vi "文本文件（将100个正弦数据以3位小数的形式写入文本文件）.vi"() -> ()   [LabVIEW 2017]
panel:
  out "写入数据":dbl[](array[numeric])
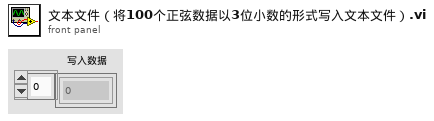
[diagram p1: front panel]
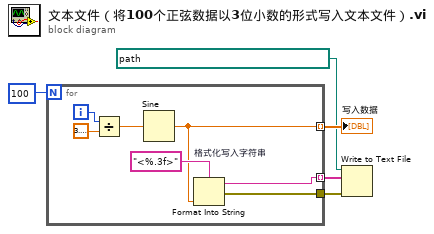
[diagram p0: block diagram]
diagram:
  n1 = for {
    N: 100 -> [_]
    tunnel: [w8] -> w4 mode=indexing
    tunnel: [w7] -> w3
    tunnel: [w6] -> w2 mode=indexing
    i -> [w12]
    n2 = Divide(x=w12, y=3.141592653589793) -> (x/y=w10:dbl)
    n3 = Sine(x=w10) -> (sin(x)=w6:dbl)
    n4 = Format Into String "格式化写入字符串"(format string="<%.3f>" ("格式字符串"), w6) -> (resulting string=w8:string, error out=w7:errorcluster)  [unwired: 2 in]
  }
  "写入数据" <- w2
  n5 = Write to Text File(file (use dialog)=path "E:/学科资料/LabView/复习/ex5-3.txt" ("文件（使用对话框）"), text=w4, error in=w3) -> ()  [unwired: 1 in, 3 out]
